vi "sensor data average.vi"(2 "Reset":bool, 3 "Data interval (s)":ext=1.0 format="%.2f", 4 "Sensor Data":T1 {"Sensor array"."scaled" format="%.2f"; "Sensor array"."voltage" format="%.4f"; "Time" format="%<%I:%M:%S%2u %p\n%m/%d/%Y>T"}) -> (0 "new data":bool, 1 "Sensor Data out":T1 {"Sensor array"."scaled" format="%.2f"; "Sensor array"."voltage" format="%.4f"; "Time" format="%<%I:%M:%S%2u %p\n%m/%d/%Y>T"})   [LabVIEW 2012]
uses:
  TCP DAQ/Sensor data.ctl
  sensor cluster.ctl
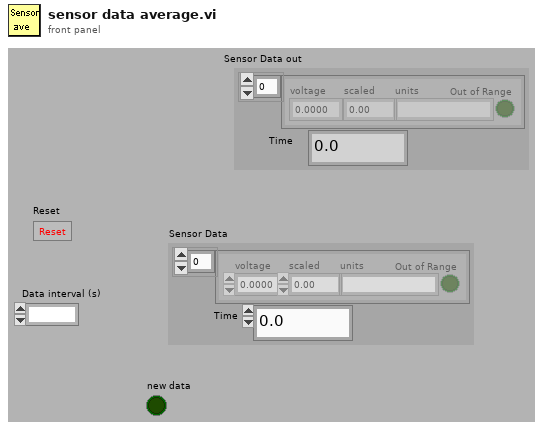
[diagram p1: front panel]
types:
  T1 = typedef "Sensor data.ctl" = cluster{" Sensor array":T2[], "Time":dbl}
  T2 = typedef "sensor cluster.ctl" = cluster{"voltage":sgl, "scaled":sgl, "units":string, "Out of Range":bool}
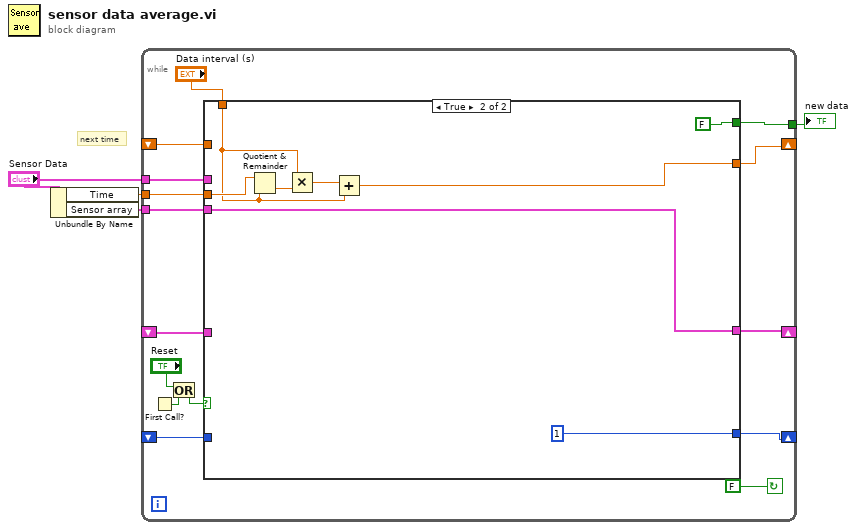
[diagram p0: block diagram]
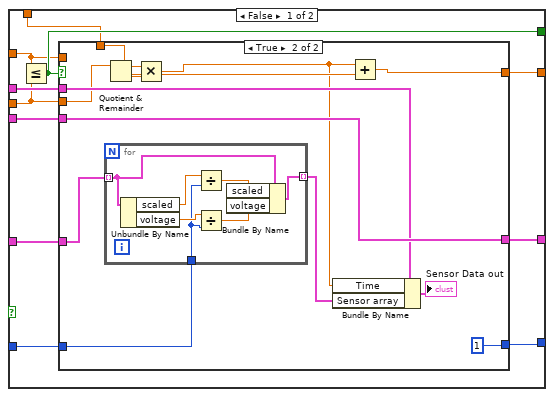
[diagram p2: hidden frame]
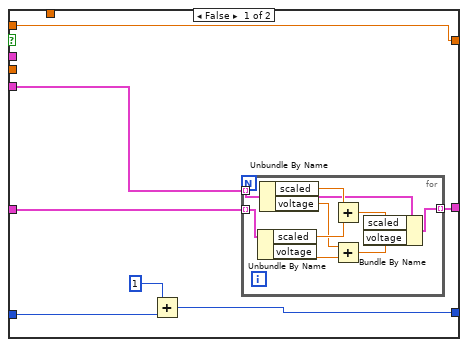
[diagram p3: hidden frame]
diagram:
  # "next time"
  n1 = Unbundle By Name("Sensor Data") -> ("Time"=w3:dbl, "Sensor array"=w1:T2[])
  n2 = while {
    shift-right: [w19] -> _
    shift-left: _ -> [w15]
    tunnel: w3 -> [w16]
    tunnel: [w17] -> w2
    shift-right: [w14] -> _
    shift-left: _ -> [w12]
    tunnel: w1 -> [w13]
    tunnel: "Sensor Data" -> [w11]
    shift-right: [w10] -> _
    shift-left: _ -> [w9]
    stop <- FALSE continue-if-true
    n3 = First Call?() -> (First Call?: T/F=w6:bool)
    n4 = Or(x="Reset", y=w6) -> (x .or. y?=w5:bool)
    n5 = case shown="True" w5 {
      tunnel: w16 -> [w20 w73]
      tunnel: [w28 w72] -> w19
      tunnel: [w30 FALSE] -> w17
      tunnel: w15 -> [w29 _]
      tunnel: [w27 w70] -> w14
      tunnel: w13 -> [w26 w70]
      tunnel: w12 -> [w25 _]
      tunnel: w11 -> [w24 _]
      tunnel: [w22 1] -> w10
      tunnel: w9 -> [w23 _]
      tunnel: "Data interval (s)" -> [w21 w67]
      frame False {
        n6 = Less Or Equal?(x=w29, y=w20) -> (x <= y?=w30:bool)
        n7 = case shown="True" w30 {
          tunnel: w29 -> [w37 _]
          tunnel: [w37 w50] -> w28
          tunnel: [w34 w58] -> w27
          tunnel: w26 -> [w36 w58]
          tunnel: w25 -> [w35 w55]
          tunnel: w24 -> [_ w57]
          tunnel: w23 -> [w32 w53]
          tunnel: [w31 1] -> w22
          tunnel: w21 -> [_ w48]
          tunnel: w20 -> [_ w51]
          frame False {
            n8 = Add(x=1, y=w32) -> (x+y=w31:i32)
            n9 = for {
              tunnel: w36 -> [w41] mode=indexing
              tunnel: w35 -> [w46] mode=indexing
              tunnel: [w38] -> w34 mode=indexing
              n10 = Unbundle By Name(w46) -> ("scaled"=w44:sgl, "voltage"=w42:sgl)
              n11 = Unbundle By Name(w41) -> ("scaled"=w45:sgl, "voltage"=w43:sgl)
              n12 = Add(x=w45, y=w44) -> (x+y=w40:sgl)
              n13 = Add(x=w43, y=w42) -> (x+y=w39:sgl)
              n14 = Bundle By Name(cluster=w41, "scaled"=w40, "voltage"=w39) -> (w38:T2)
            }
          }
          frame True {
            n15 = for {
              tunnel: w55 -> [w59] mode=indexing
              tunnel: [w63] -> w54 mode=indexing
              tunnel: w53 -> [w60]
              n16 = Unbundle By Name(w59) -> ("scaled"=w61:sgl, "voltage"=w62:sgl)
              n17 = Divide(x=w61, y=w60) -> (x/y=w65:sgl)
              n18 = Divide(x=w62, y=w60) -> (x/y=w64:sgl)
              n19 = Bundle By Name(cluster=w59, "scaled"=w65, "voltage"=w64) -> (w63:T2)
            }
            n20 = Quotient & Remainder(x=w51, y=w48) -> (floor(x/y)=w49:ext)  [unwired: 1 out]
            n21 = Multiply(x=w48, y=w49) -> (x*y=w47:ext)
            n22 = Bundle By Name(cluster=w57, "Time"=w47, "Sensor array"=w54) -> (→"Sensor Data out":T1)
            n23 = Add(x=w47, y=w48) -> (x+y=w50:ext)
          }
        }
      }
      frame True {
        n24 = Quotient & Remainder(x=w73, y=w67) -> (floor(x/y)=w68:ext)  [unwired: 1 out]
        n25 = Multiply(x=w67, y=w68) -> (x*y=w66:ext)
        n26 = Add(x=w66, y=w67) -> (x+y=w72:ext)
      }
    }
  }
  "new data" <- w2
